vi "Read Measurement.vi"(0 "VISA resource name":refnum<visa-resource-name>, 11 "error in (no error)":errorcluster) -> (3 "primary\ncomparison result":u16, 4 "VISA resource name out":refnum<visa-resource-name>, 6 "status":u16, 8 "primary reading":dbl format="%.5e", 10 "secondary reading":dbl format="%.5e", 14 "secondary\ncomparison result":u16, 15 "error out":errorcluster)   [LabVIEW 2016, in "Agilent 4263X.lvlib"]
doc: "This VI reads the primary and secondary measurements currently active. See the Config Measurement VI and Config Measurement Parameters VI for configuring of measurement type.\n\n*NOTE: The instrument must have been previously triggered before this VI can be properly executed."
uses:
  <instrlib>/Agilent 4263X/Agilent 4263X.lvlib
panel:
  # "*NOTE:  The instrument must have been\npreviously triggered before this VI can be\nproperly executed."
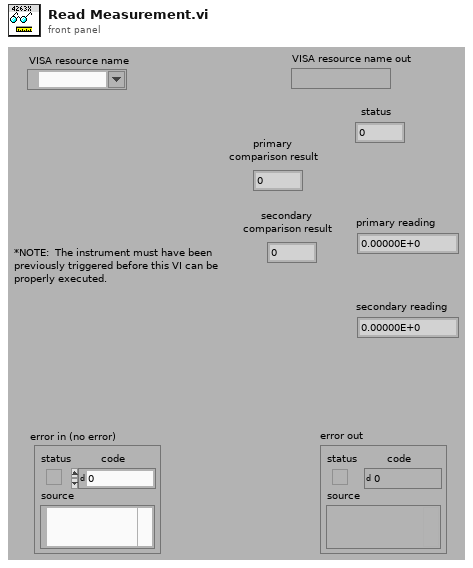
[diagram p1: front panel]
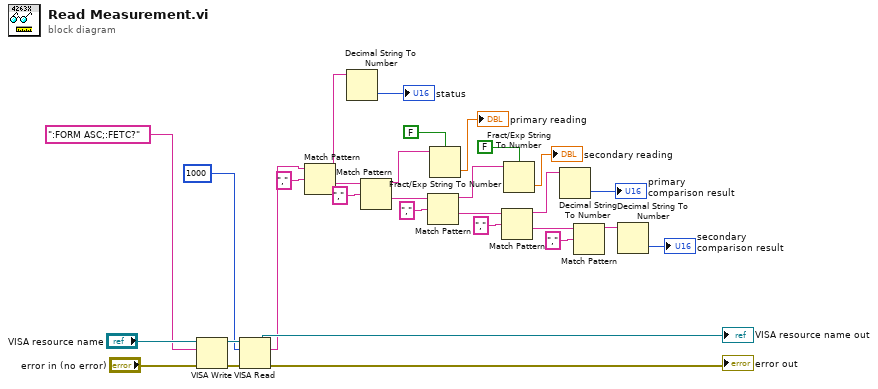
[diagram p0: block diagram]
diagram:
  n1 = VISA Write(VISA resource name="VISA resource name", write buffer=":FORM ASC;:FETC?", error in (no error)="error in (no error)") -> (VISA resource name out=w30:refnum<visa-resource-name>, error out=w29:errorcluster)  [unwired: 1 out]
  n2 = VISA Read(VISA resource name=w30, byte count=1000, error in (no error)=w29) -> (VISA resource name out=→"VISA resource name out":refnum<visa-resource-name>, read buffer=w9:string, error out=→"error out":errorcluster)  [unwired: 1 out]
  n3 = Match Pattern(string=w9, regular expression=",") -> (before substring=w12:string, after substring=w10:string)  [unwired: 1 in, 2 out]
  n4 = Decimal String To Number(string=w12) -> (number=→"status":i32)  [unwired: 2 in, 1 out]
  n5 = Match Pattern(string=w10, regular expression=",") -> (before substring=w22:string, after substring=w16:string)  [unwired: 1 in, 2 out]
  n6 = Match Pattern(string=w16, regular expression=",") -> (before substring=w14:string, after substring=w13:string)  [unwired: 1 in, 2 out]
  n7 = Fract/Exp String To Number(use system decimal point (T)=FALSE, string=w22) -> (number=→"primary reading":dbl)  [unwired: 2 in, 1 out]
  n8 = Match Pattern(string=w13, regular expression=",") -> (before substring=w21:string, after substring=w5:string)  [unwired: 1 in, 2 out]
  n9 = Fract/Exp String To Number(use system decimal point (T)=FALSE, string=w14) -> (number=→"secondary reading":dbl)  [unwired: 2 in, 1 out]
  n10 = Decimal String To Number(string=w21) -> (number=→"primary\ncomparison result":i32)  [unwired: 2 in, 1 out]
  n11 = Match Pattern(string=w5, regular expression=",") -> (before substring=w4:string)  [unwired: 1 in, 3 out]
  n12 = Decimal String To Number(string=w4) -> (number=→"secondary\ncomparison result":i32)  [unwired: 2 in, 1 out]
